vi "Scaled noise.vi"(1 "Fraction":dbl, 2 "Input":dbl) -> (0 "Output with noise":dbl)   [LabVIEW 2018]
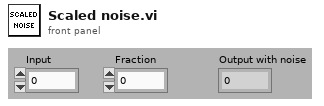
[diagram p1: front panel]
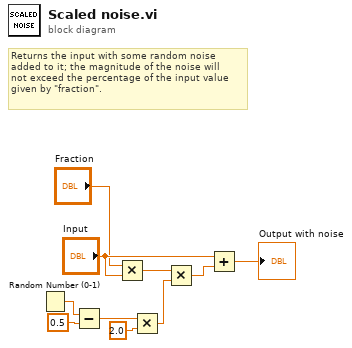
[diagram p0: block diagram]
diagram:
  # "Returns the input with some random noise\nadded to it; the magnitude of the noise will\nnot exceed the percentage of the input value\ngiven by \"fraction\"."
  n1 = Random Number (0-1)() -> (number: 0 to 1=w5:dbl)
  n2 = Subtract(x=w5, y=0.5) -> (x-y=w3:dbl)
  n3 = Multiply(x="Fraction", y="Input") -> (x*y=w6:dbl)
  n4 = Multiply(x=w3, y=2.0) -> (x*y=w1:dbl)
  n5 = Multiply(x=w6, y=w1) -> (x*y=w8:dbl)
  n6 = Add(x="Input", y=w8) -> (x+y=→"Output with noise":dbl)
